vi "sweep_gate_wait_for_meas.vi"() -> ()   [LabVIEW 2024]
uses:
  <vilib>/Analysis/1siggen.llb/Ramp Pattern by Delta.vi
  C:/Users/Public/OneDrive/Desktop/Keithley_2450_2470_1_4_0_LV2015_NewReadme2_2450-LV2015-1.4.0/Keithley 2450/Keithley 2450.lvlib
  <vilib>/Analysis/NI_AALBase.lvlib
panel:
  in  "Loop?":bool=TRUE
  out "Current voltage":dbl
  in  "V stepsize":dbl
  in  "start V":dbl
  in  "end V":dbl
  in  "Wait time (ms)":i32=2000
  in  "Limit Reached 2":bool
  in  "Current Compliance Limit (0.1)":dbl=5e-08
  in  "Max Elapsed time (s)":u32=1
  in  "Measure Interval (ms)":u32=100
  out "Current":dbl caption="Measured Current (A)"
  in  "stop":bool
  out "XY Graph":cluster{dbl[], dbl[]}(graph)
  in  "error in (no error)":errorcluster
  in  "VISA resource name 2":refnum<visa-resource-name>="GPIB0::18::INSTR"
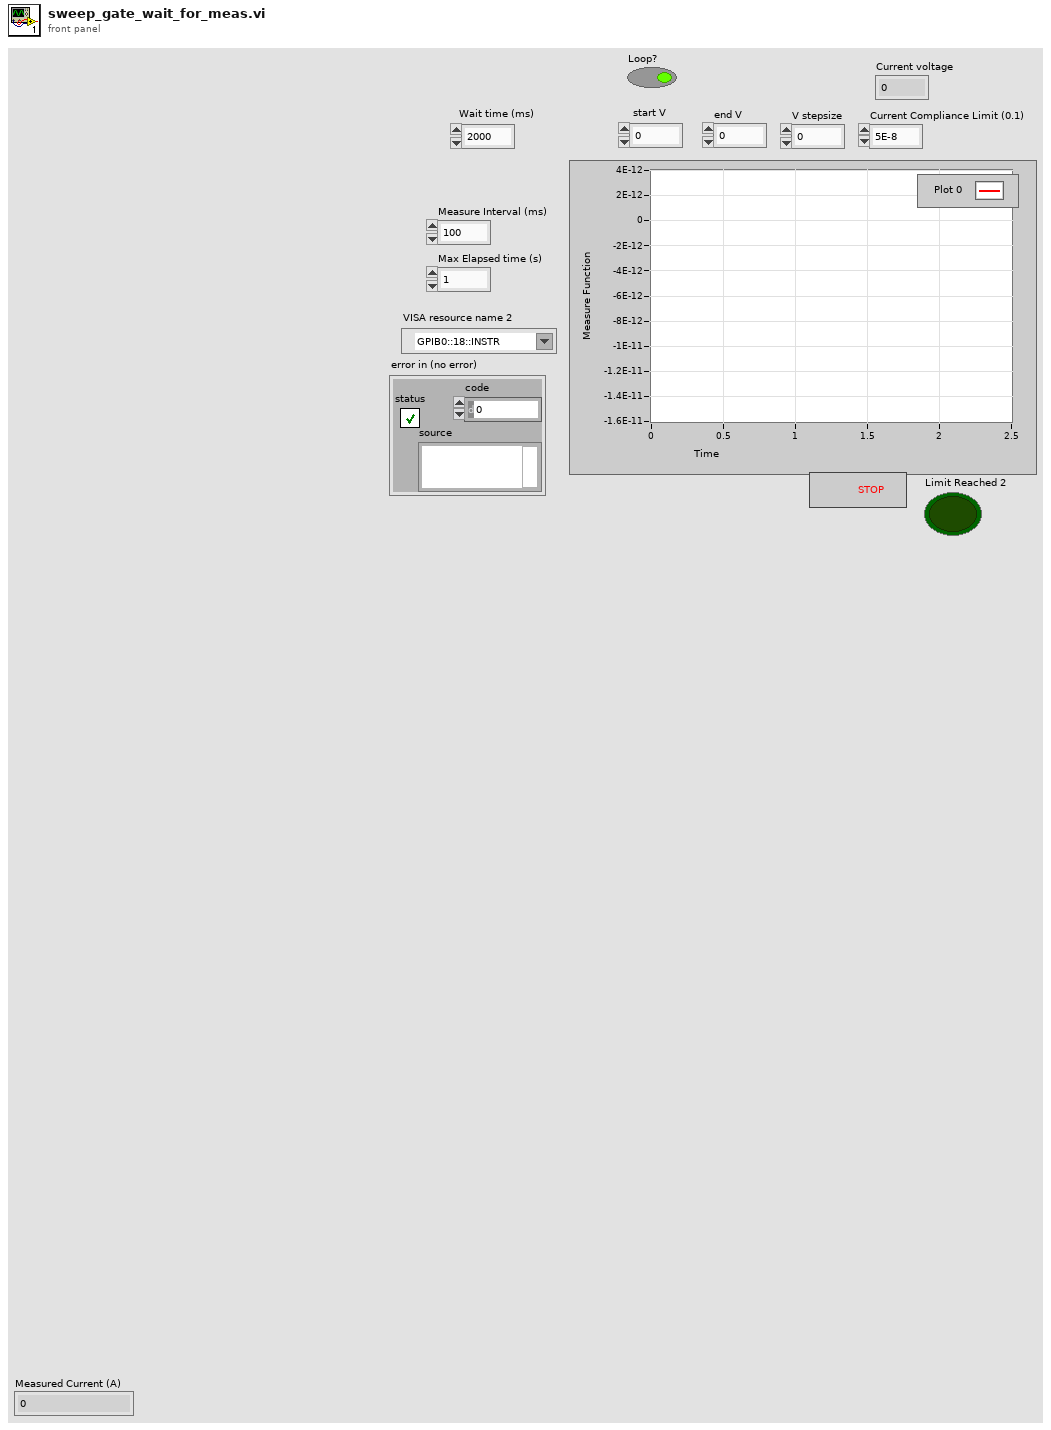
[diagram p1: front panel]
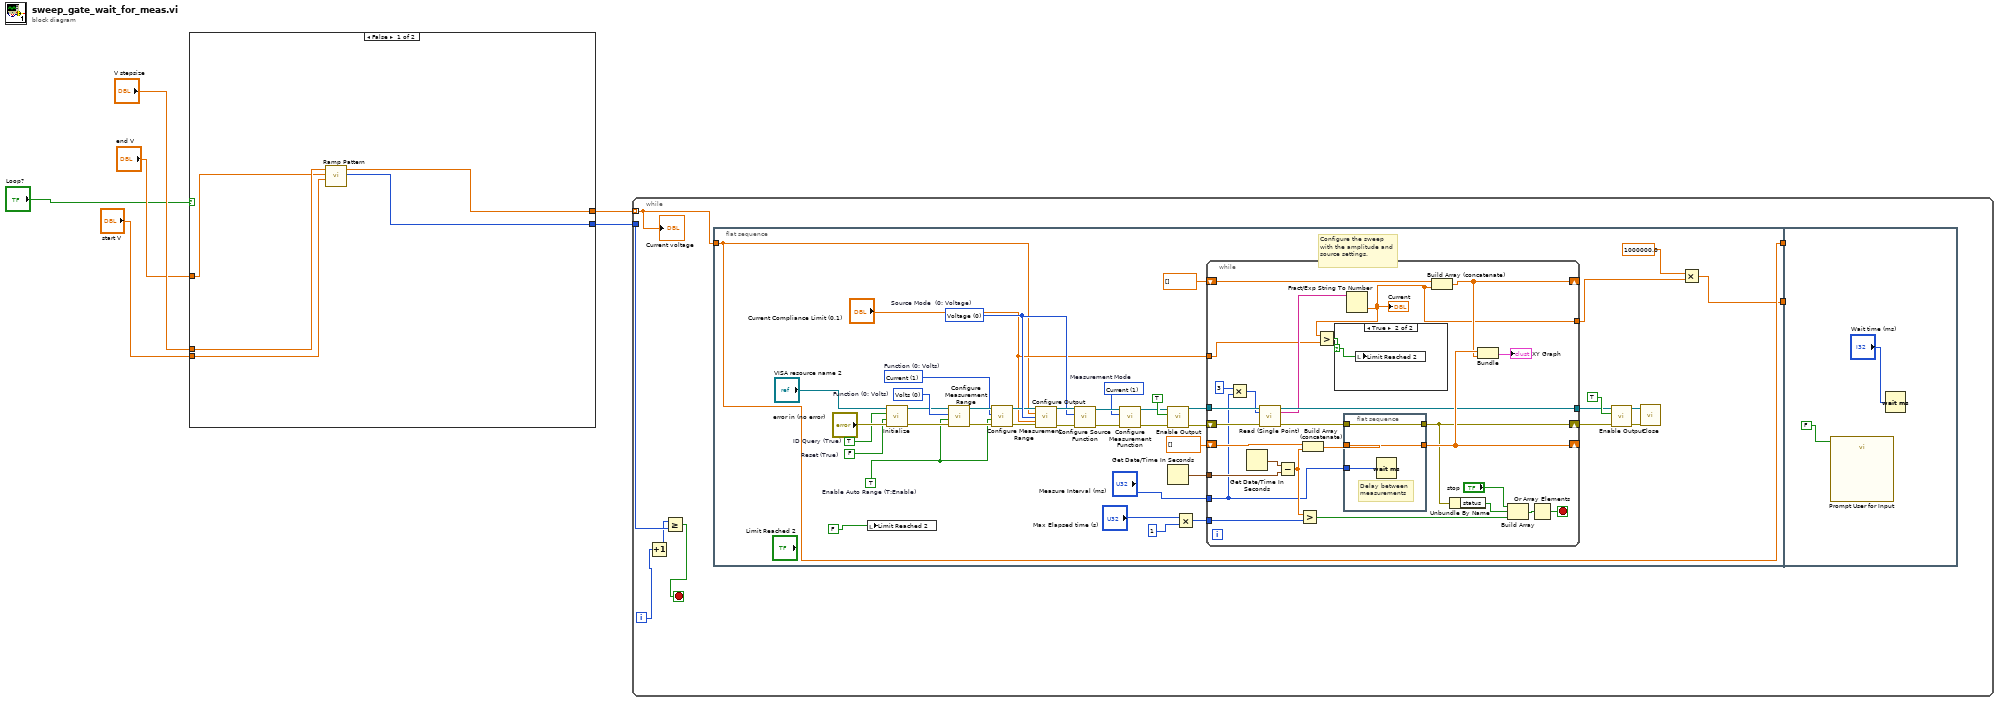
[diagram p0: block diagram]
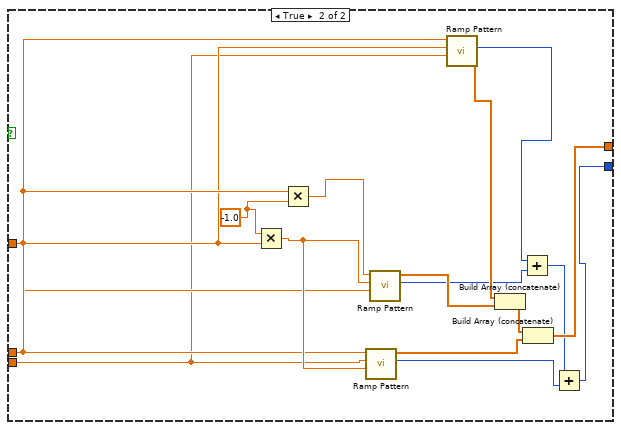
[diagram p2: hidden frame]
diagram:
  n1 = case shown="False" "Loop?" {
    tunnel: [w7 w12] -> w6
    tunnel: [w8 w15] -> w5
    tunnel: "V stepsize" -> [w11 w20]
    tunnel: "end V" -> [w10 w19]
    tunnel: "start V" -> [w9 w18]
    frame False {
      n2 = call-poly <vilib>:"Ramp Pattern.vi"("start"=w9, "end"=w10, "delta"=w11) -> ("samples"=w7:i32, "Ramp Pattern"=w8:dbl[])  [unwired: 6 in, 1 out]
    }
    frame True {
      w22 = -1.0
      n3 = Multiply(x=w22, y=w19) -> (x*y=w21:dbl)
      n4 = Multiply(x=w20, y=w22) -> (x*y=w26:dbl)
      n5 = call-poly <vilib>:"Ramp Pattern.vi"("start"=w21, "end"=w18, "delta"=w20) -> ("samples"=w13:i32, "Ramp Pattern"=w16:dbl[])  [unwired: 6 in, 1 out]
      n6 = call-poly <vilib>:"Ramp Pattern.vi"("start"=w19, "end"=w21, "delta"=w26) -> ("samples"=w23:i32, "Ramp Pattern"=w27:dbl[])  [unwired: 6 in, 1 out]
      n7 = call-poly <vilib>:"Ramp Pattern.vi"("start"=w18, "end"=w19, "delta"=w20) -> ("samples"=w24:i32, "Ramp Pattern"=w25:dbl[])  [unwired: 6 in, 1 out]
      n8 = Build Array (concatenate)(w25, w27) -> (w17:dbl[])
      n9 = Add(x=w24, y=w23) -> (x+y=w14:i32)
      n10 = Build Array (concatenate)(w17, w16) -> (w15:dbl[])
      n11 = Add(x=w14, y=w13) -> (x+y=w12:i32)
    }
  }
  n12 = while {
    tunnel: w5 -> [w32] mode=indexing
    tunnel: w6 -> [w34]
    i -> [w31]
    stop <- w33 stop-if-true
    n13 = Increment(x=w31) -> (x+1=w30:i32)
    n14 = Greater Or Equal?(x=w30, y=w34) -> (x >= y?=w33:bool)
    n15 = flat-sequence {
      tunnel: w32 -> [w38]
      tunnel: [w37] -> w29
      tunnel: [w38] -> w28
      tunnel: w29 -> [_]
      tunnel: w28 -> [_]
      frame #0 {
        w61 = u16 0 items=["Voltage", "Current"]  # Source Mode  (0: Voltage)
        w42 = u16 1 items=["Volts", "Current", "Auto Resistance", "Manual Resistance", "Digitize Voltage", "Digitize Current"]  # Measurement Mode
        w57 = TRUE  # Enable Auto Range (T:Enable)
        w66 = u16 1 items=["Volts", "Current", "Resistance"]  # Function (0: Volts)
        w67 = u16 0 items=["Volts", "Current", "Resistance"]  # Function (0: Volts)
        w59 = FALSE  # Reset (True)
        w58 = TRUE  # ID Query (True)
        # "Configure the sweep with the amplitude and source settings."
        n16 = local write "Limit Reached 2"(FALSE) -> ()
        n17 = call "Initialize.vi"("error in (no error)"="error in (no error)", "Reset (True)"=w59, "ID Query (True)"=w58, "VISA resource name"="VISA resource name 2") -> ("error out"=w64:errorcluster, "VISA resource name out"=w65:refnum<visa-resource-name>)  [unwired: 6 in]
        n18 = call "Configure Measurement Range.vi"("error in (no error)"=w64, "Enable Auto Range (T:Enable)"=w57, "Function (0: Volts)"=w67, "VISA resource name"=w65) -> ("error out"=w68:errorcluster, "VISA resource name out"=w69:refnum<visa-resource-name>)  [unwired: 6 in]
        n19 = call "Configure Measurement Range.vi"("error in (no error)"=w68, "Enable Auto Range (T:Enable)"=w57, "Function (0: Volts)"=w66, "VISA resource name"=w69) -> ("error out"=w44:errorcluster, "VISA resource name out"=w43:refnum<visa-resource-name>)  [unwired: 6 in]
        n20 = call "Configure Output.vi"("VISA resource name"=w43, "Source Level (0)"=w38, "Source Mode  (0: Voltage)"=w61, "Source Limit Level (0.1)"="Current Compliance Limit (0.1)", "error in (no error)"=w44) -> ("VISA resource name out"=w63:refnum<visa-resource-name>, "error out"=w62:errorcluster)  [unwired: 9 in]
        n21 = call "Configure Source Function.vi"("error in (no error)"=w62, "Function (0: Volts)"=w61, "VISA resource name"=w63) -> ("error out"=w56:errorcluster, "VISA resource name out"=w55:refnum<visa-resource-name>)  [unwired: 7 in]
        n22 = call "Configure Measurement Function.vi"("error in (no error)"=w56, "Function (0: Volts)"=w42, "VISA resource name"=w55) -> ("error out"=w52:errorcluster, "VISA resource name out"=w51:refnum<visa-resource-name>)  [unwired: 7 in]
        n23 = Get Date/Time In Seconds() -> (seconds since 1Jan1904=w76:timestamp)
        n24 = call "Enable Output.vi"("error in (no error)"=w52, "Enable Output (T: Enable)"=TRUE, "VISA resource name"=w51) -> ("error out"=w53:errorcluster, "VISA resource name out"=w45:refnum<visa-resource-name>)  [unwired: 7 in]
        n25 = Multiply(x="Max Elapsed time (s)", y=u32 1) -> (x*y=w70:u32)
        n26 = while {
          shift-right: [w85] -> w47
          shift-left: w53 -> [w88]
          tunnel: w76 -> [w102]
          shift-right: [w96] -> _
          shift-left: dbl[] [] -> [w101]
          shift-right: [w95] -> _
          shift-left: dbl[] [] -> [w100]
          tunnel: "Measure Interval (ms)" -> [w83]
          tunnel: w70 -> [w92]
          tunnel: [w81] -> w46
          tunnel: w45 -> [w86]
          tunnel: "Current Compliance Limit (0.1)" -> [w79]
          tunnel: [w77] -> w35
          stop <- w99 stop-if-true
          n27 = Multiply(x=u32 3, y=w83) -> (x*y=w84:u32)
          n28 = Get Date/Time In Seconds() -> (seconds since 1Jan1904=w103:timestamp)
          n29 = call "Read (Single Point).vi"("VISA resource name"=w86, "Timeout (10000 ms)"=w84, "error in (no error)"=w88) -> ("VISA resource name out"=w81:refnum<visa-resource-name>, "Data out"=w80:string, "error out"=w87:errorcluster)  [unwired: 10 in]
          n30 = Subtract(x=w103, y=w102) -> (x-y=w93:dbl)
          n31 = Greater?(x=w93, y=w92) -> (0:w89:bool)
          n32 = Build Array (concatenate)(w101, w93) -> (w97:dbl[])
          n33 = flat-sequence {
            tunnel: w97 -> [w107]
            tunnel: [w107] -> w96
            tunnel: w83 -> [w106]
            tunnel: w87 -> [w105]
            tunnel: [w105] -> w85
            frame #0 {
              # "Delay between\nmeasurements"
              n34 = Wait (ms)(milliseconds to wait=w106) -> ()  [unwired: 1 out]
            }
          }
          n35 = Fract/Exp String To Number(string=w80) -> (number=w77:dbl)  [unwired: 3 in, 1 out]
          "Current" <- w77
          n36 = Greater?(x=w77, y=w79) -> (0:w78:bool)
          n37 = case shown="True" w78 {
            selector: w78 -> [_ w104]
            frame False {
            }
            frame True {
              n38 = local write "Limit Reached 2"(w104) -> ()
            }
          }
          n39 = Build Array (concatenate)(w100, w77) -> (w95:dbl[])
          n40 = Unbundle By Name(w85) -> ("status"=w90:bool)
          n41 = Bundle(w96, w95) -> (→"XY Graph":cluster{dbl[], dbl[]})  [unwired: 1 in]
          n42 = Build Array("stop", w90, w89) -> (w98:bool[])
          n43 = Or Array Elements(Boolean array=w98) -> (logical OR=w99:bool)
        }
        n44 = call "Enable Output.vi"("error in (no error)"=w47, "Enable Output (T: Enable)"=TRUE, "VISA resource name"=w46) -> ("error out"=w48:errorcluster, "VISA resource name out"=w49:refnum<visa-resource-name>)  [unwired: 7 in]
        n45 = call "Close.vi"("error in (no error)"=w48, "VISA resource name"=w49) -> ()  [unwired: 9 in, 1 out]
        n46 = Multiply(x=1000000.0, y=w35) -> (x*y=w37:dbl)
      }
      frame #1 {
        n47 = call "Prompt User for Input"("Enable"=FALSE) -> ()  [unwired: 17 in, 2 out]
        n48 = Wait (ms)(milliseconds to wait="Wait time (ms)") -> ()  [unwired: 1 out]
      }
    }
    "Current voltage" <- w32
  }
